vi "Create Color Array.vi"(11 "RGB in":u8[](array[numeric])) -> (2 "U32 color":u32[](array[numeric]))   [LabVIEW 2020, in "lv_icon.lvlib"]
doc: "Create a color array based on an RGB input"
uses:
  <vilib>/LabVIEW Icon API/lv_icon/lv_icon.lvlib
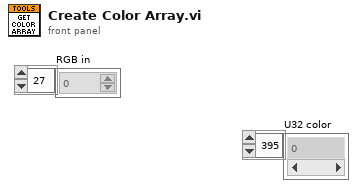
[diagram p1: front panel]
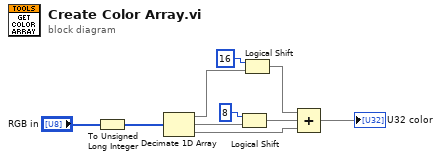
[diagram p0: block diagram]
diagram:
  n1 = To Unsigned Long Integer(number="RGB in") -> (unsigned 32bit integer=w5:u32[])
  n2 = Decimate 1D Array(w5) -> (w9:u32[], w3:u32[], w8:u32[])
  n3 = Logical Shift(y=i16 8, x=w3) -> (x << y=w2:u32[])
  n4 = Logical Shift(y=i16 16, x=w9) -> (x << y=w7:u32[])
  n5 = Compound Arithmetic op=ADD(w7, w2, w8) -> (→"U32 color":u32[])
